vi "client.vi"() -> ()   [LabVIEW 2018]
panel:
  in  "Attacked Audio File Path 2":path
  out "Attacked Audio":waveform(dbl)[](graph)
  in  "Upload":bool
  in  "Quit":bool
  in  "Original Audio File Path":path
  out "Original Audio":waveform(dbl)[](graph)
  in  "Port Number":u16
  in  "IP Address":string
  in  "Target":string(combo)
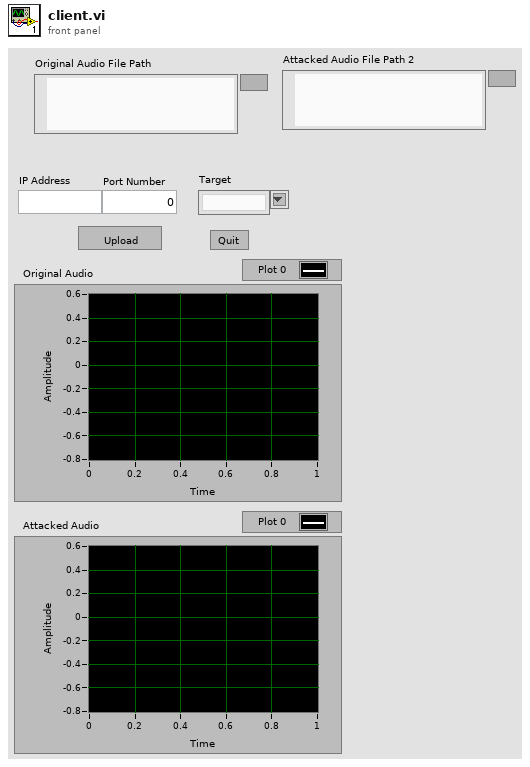
[diagram p1: front panel]
types:
  T1 = enum16{"open", "replace", "create", "open or create", "replace or create", "replace or create with confirmation"}
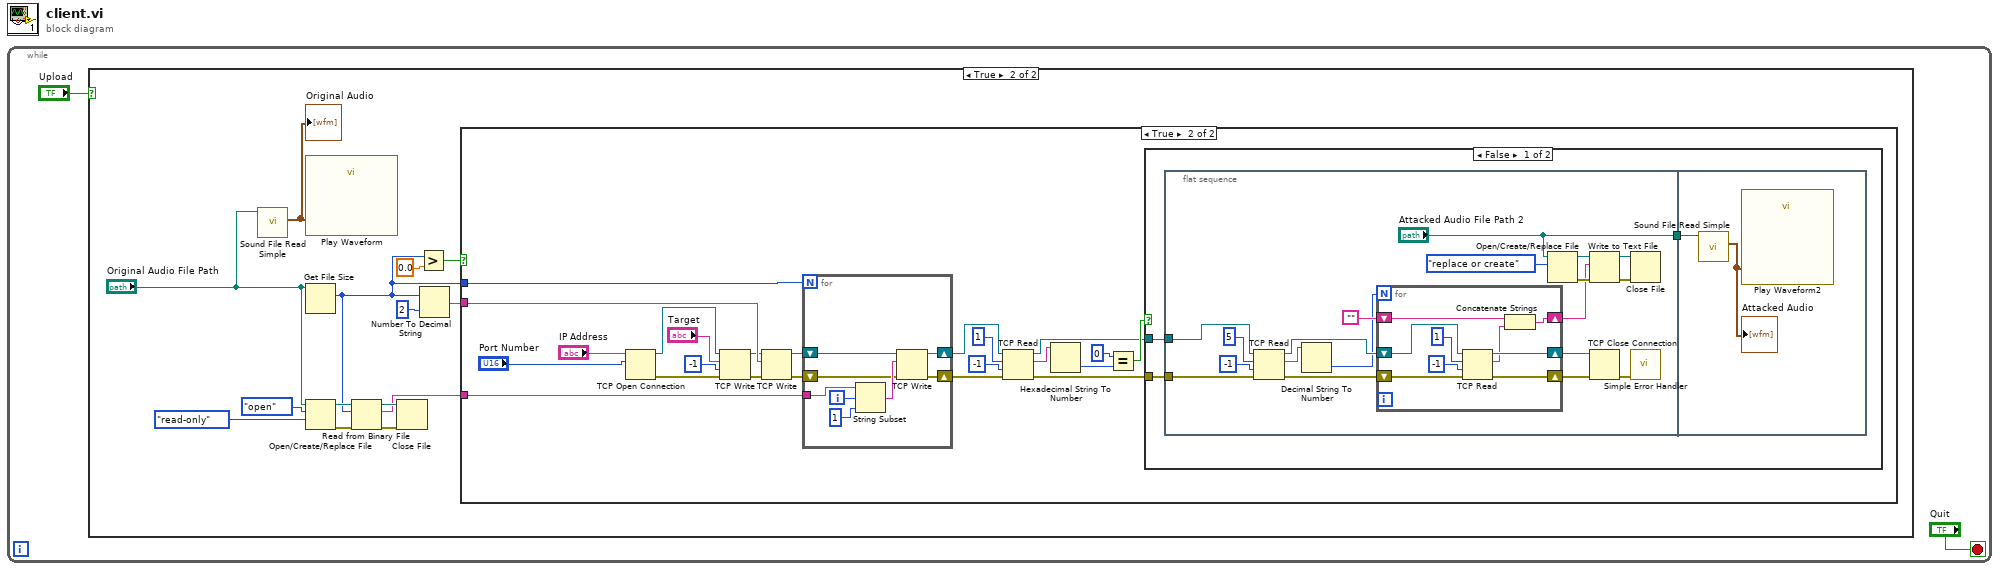
[diagram p0: block diagram]
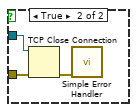
[diagram p4: hidden frame]
diagram:
  n1 = while {
    stop <- "Quit" stop-if-true
    n2 = case shown="True" "Upload" {
      frame False {
      }
      frame True {
        n3 = call <vilib>:"Sound File Read Simple.vi"("path"="Original Audio File Path") -> ("data"=w16:waveform(dbl)[])  [unwired: 7 in, 3 out]
        "Original Audio" <- w16
        n4 = call "Play Waveform"("Data"=w16) -> ()  [unwired: 18 in, 1 out]
        n5 = Get File Size(file="Original Audio File Path") -> (size (in bytes)=w3:i64)  [unwired: 1 in, 2 out]
        n6 = Open/Create/Replace File(file path (use dialog)="Original Audio File Path", operation (0:open)=T1."open", access (0:read/write)=enum16{"read/write", "read-only", "write-only"}."read-only") -> (refnum out=w12:refnum<file>, error out=w11:errorcluster)  [unwired: 3 in, 1 out]
        n7 = Read from Binary File(8:w11, 10:w3, 11:w12) -> (0:w9:errorcluster, 2:w4:string, 3:w10:refnum<file>)  [unwired: 3 in, 1 out]
        n8 = Close File(refnum=w10, error in=w9) -> ()  [unwired: 2 out]
        n9 = Greater?(x=w3, y=0.0) -> (0:w7:bool)
        n10 = Number To Decimal String(number=w3, width (-)=i16 2) -> (decimal integer string=w5:string)
        n11 = case shown="True" w7 {
          tunnel: w5 -> [_ w33]
          tunnel: w3 -> [_ w32]
          tunnel: w4 -> [_ w27]
          frame False {
          }
          frame True {
            n12 = TCP Open Connection(address="IP Address", remote port or service name="Port Number") -> (connection ID=w36:refnum<k5>, error out=w37:errorcluster)  [unwired: 3 in]
            n13 = TCP Write(connection ID=w36, data in="Target", error in (no error)=w37, 9:-1 ("timeout ms (25000)")) -> (connection ID out=w31:refnum<k5>, error out=w30:errorcluster)  [unwired: 1 out]
            n14 = TCP Write(connection ID=w31, data in=w33, error in (no error)=w30) -> (connection ID out=w29:refnum<k5>, error out=w28:errorcluster)  [unwired: 1 in, 1 out]
            n15 = for {
              N: w32 -> [_]
              shift-right: [w79] -> w26
              shift-left: w29 -> [w82]
              shift-right: [w78] -> w25
              shift-left: w28 -> [w81]
              tunnel: w27 -> [w80]
              i -> [w77]
              n16 = String Subset(string=w80, offset (0)=w77, length (rest)=1 ("y")) -> (substring=w83:string)
              n17 = TCP Write(connection ID=w82, data in=w83, error in (no error)=w81) -> (connection ID out=w79:refnum<k5>, error out=w78:errorcluster)  [unwired: 1 in, 1 out]
            }
            n18 = TCP Read(connection ID=w26, bytes to read=1, error in (no error)=w25, 9:-1 ("timeout ms (25000)")) -> (connection ID out=w18:refnum<k5>, data out=w22:string, error out=w17:errorcluster)  [unwired: 1 in]
            n19 = Hexadecimal String To Number(string=w22) -> (number=w20:u32)  [unwired: 2 in, 1 out]
            n20 = Equal?(x=u32 0, y=w20) -> (x = y?=w21:bool)
            n21 = case shown="False" w21 {
              tunnel: w18 -> [w42 w74]
              tunnel: w17 -> [w41 w73]
              frame False {
                n22 = flat-sequence {
                  tunnel: w42 -> [w61]
                  tunnel: w41 -> [w58]
                  tunnel: ["Attacked Audio File Path 2"] -> w40
                  tunnel: w40 -> [w72]
                  frame #0 {
                    n23 = TCP Read(connection ID=w61, bytes to read=5, error in (no error)=w58, 9:-1 ("timeout ms (25000)")) -> (connection ID out=w55:refnum<k5>, data out=w51:string, error out=w56:errorcluster)  [unwired: 1 in]
                    n24 = Decimal String To Number(string=w51) -> (number=w50:i32)  [unwired: 2 in, 1 out]
                    n25 = for {
                      N: w50 -> [_]
                      shift-right: [w67] -> w53
                      shift-left: w55 -> [w70]
                      shift-right: [w68] -> w54
                      shift-left: w56 -> [w69]
                      shift-right: [w65] -> w47
                      shift-left: "" -> [w64]
                      n26 = TCP Read(connection ID=w70, bytes to read=1, error in (no error)=w69, 9:-1 ("timeout ms (25000)")) -> (connection ID out=w67:refnum<k5>, data out=w62:string, error out=w68:errorcluster)  [unwired: 1 in]
                      n27 = Concatenate Strings(w64, w62) -> (w65:string)
                    }
                    n28 = Open/Create/Replace File(file path (use dialog)="Attacked Audio File Path 2", operation (0:open)=T1."replace or create") -> (refnum out=w49:refnum<file>, error out=w48:errorcluster)  [unwired: 4 in, 1 out]
                    n29 = Write to Text File(file (use dialog)=w49, text=w47, error in=w48) -> (refnum out=w44:refnum<file>, error out=w46:errorcluster)  [unwired: 1 in, 1 out]
                    n30 = TCP Close Connection(connection ID=w53, error in (no error)=w54) -> (error out=w57:errorcluster)  [unwired: 1 in, 1 out]
                    n31 = Close File(refnum=w44, error in=w46) -> ()  [unwired: 2 out]
                    n32 = call <vilib>:"Simple Error Handler.vi"("error in (no error)"=w57) -> ()  [unwired: 4 in, 5 out]
                  }
                  frame #1 {
                    n33 = call <vilib>:"Sound File Read Simple.vi"("path"=w72) -> ("data"=w71:waveform(dbl)[])  [unwired: 7 in, 3 out]
                    "Attacked Audio" <- w71
                    n34 = call "Play Waveform2"("Data"=w71) -> ()  [unwired: 18 in, 1 out]
                  }
                }
              }
              frame True {
                n35 = TCP Close Connection(connection ID=w74, error in (no error)=w73) -> (error out=w75:errorcluster)  [unwired: 1 in, 1 out]
                n36 = call <vilib>:"Simple Error Handler.vi"("error in (no error)"=w75) -> ()  [unwired: 4 in, 5 out]
              }
            }
          }
        }
      }
    }
  }
